vi "Build Enable Cluster.vi"(1 "Enable Array":dbl[](array[numeric])) -> (0 "Enable Flag Cluster":T1)   [LabVIEW 2015, in "Fuel Injection Addon Engine.lvlib"]
uses:
  Fuel Injection Addon Engine.lvlib
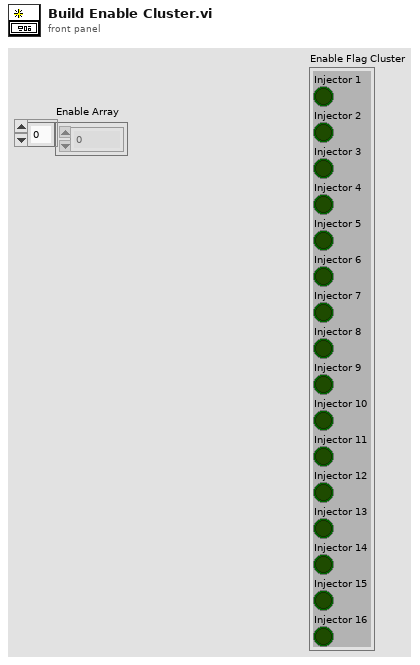
[diagram p1: front panel]
types:
  T1 = cluster{"Injector 1":bool, "Injector 2":bool, "Injector 3":bool, "Injector 4":bool, "Injector 5":bool, "Injector 6":bool, "Injector 7":bool, "Injector 8":bool, "Injector 9":bool, "Injector 10":bool, "Injector 11":bool, "Injector 12":bool, "Injector 13":bool, "Injector 14":bool, "Injector 15":bool, "Injector 16":bool}
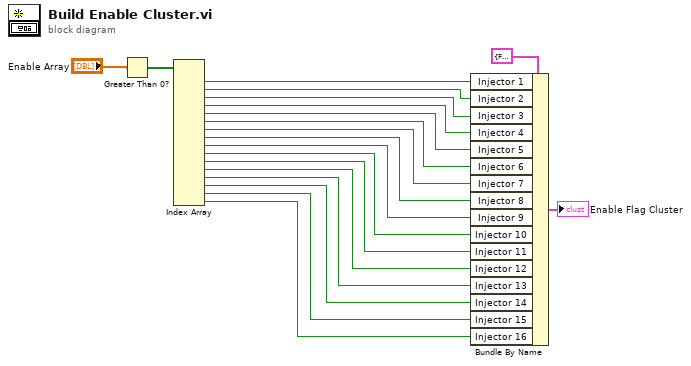
[diagram p0: block diagram]
diagram:
  n1 = Greater Than 0?(x="Enable Array") -> (x > 0?=w1:bool[])
  n2 = Index Array(array=w1) -> (element #1=w19:bool, element #2=w18:bool, element #3=w17:bool, element #4=w16:bool, element #5=w15:bool, element #6=w14:bool, element #7=w13:bool, element #8=w12:bool, element #9=w11:bool, element #10=w10:bool, element #11=w9:bool, element #12=w8:bool, element #13=w7:bool, element #14=w6:bool, element #15=w5:bool, element #16=w4:bool)  [unwired: 16 in]
  n3 = Bundle By Name(cluster=T1 {"Injector 1"=FALSE, "Injector 2"=FALSE, "Injector 3"=FALSE, "Injector 4"=FALSE, "Injector 5"=FALSE, "Injector 6"=FALSE, "Injector 7"=FALSE, "Injector 8"=FALSE, "Injector 9"=FALSE, "Injector 10"=FALSE, "Injector 11"=FALSE, "Injector 12"=FALSE, "Injector 13"=FALSE, "Injector 14"=FALSE, "Injector 15"=FALSE, "Injector 16"=FALSE} ("Enable Acquisition Cluster"), "Injector 1"=w19, "Injector 2"=w18, "Injector 3"=w17, "Injector 4"=w16, "Injector 5"=w15, "Injector 6"=w14, "Injector 7"=w13, "Injector 8"=w12, "Injector 9"=w11, "Injector 10"=w10, "Injector 11"=w9, "Injector 12"=w8, "Injector 13"=w7, "Injector 14"=w6, "Injector 15"=w5, "Injector 16"=w4) -> (→"Enable Flag Cluster":T1)
